vi "Setup file output channels.vi"(8 "error in":errorcluster, 9 "Sampling data":T1 {"Channels"."Hi cutoff" items=["500"=500.0, "1k"=1000.0, "5k"=5000.0, "10k"=10000.0, "20k"=20000.0]; "Channels"."Lo cutoff" items=["0.1"=0.1, "1"=1.0, "10"=10.0, "100"=100.0, "300"=300.0]; "Channels"."Gain" items=["x100"=100, "x1000"=1000, "x10000"=10000]}, 11 "file ref in":T3 format="%.0x") -> (0 "error out":errorcluster, 1 "Sampling data out":T1 {"Channels"."Hi cutoff" items=["500"=500.0, "1k"=1000.0, "5k"=5000.0, "10k"=10000.0, "20k"=20000.0]; "Channels"."Lo cutoff" items=["0.1"=0.1, "1"=1.0, "10"=10.0, "100"=100.0, "300"=300.0]; "Channels"."Gain" items=["x100"=100, "x1000"=1000, "x10000"=10000]}, 2 "dset ref":i32, 3 "file ref out":T3 format="%.0x", 4 "cmd dset out":i32)   [LabVIEW 2012]
uses:
  <vilib>/addons/h5labview2/base/hid_t.ctl
  Sampling info.ctl
  Channel.ctl
  Create HDF5 chunked dataset (2D).vi
  <vilib>/addons/h5labview2/base/H5Equery.vi
  <vilib>/addons/h5labview2/attrib/H5Awrite.llb/H5Awrite.xnode
  <vilib>/addons/h5labview2/group/H5G.lvlib
  <vilib>/addons/h5labview2/h5labview32.dll
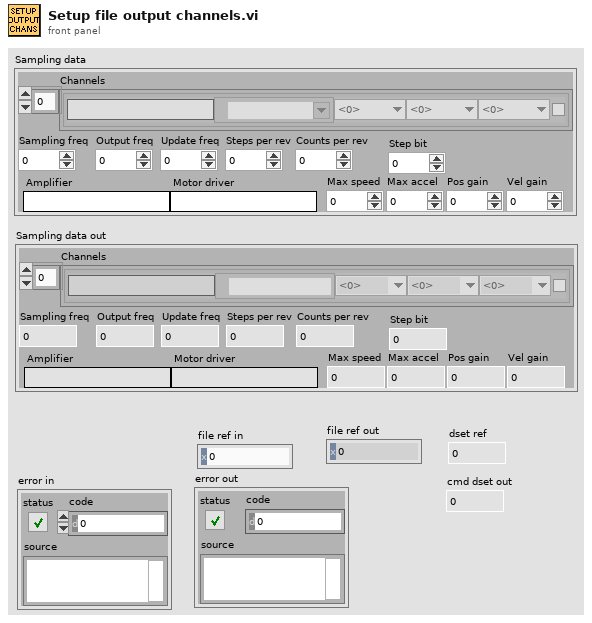
[diagram p1: front panel]
types:
  T1 = typedef "Sampling info.ctl" = cluster{"Channels":T2[], "Sampling freq":i32, "Output freq":i32, "Update freq":i32, "Steps per rev":i32, "Counts per rev":i32, "Amplifier":string, "Motor driver":string, "Step bit":u8, "Max speed":dbl, "Max accel":dbl, "Pos gain":dbl, "Vel gain":dbl}
  T2 = typedef "Channel.ctl" = cluster{"Name":string, "Chan":tag, "Gain":u16, "Lo cutoff":dbl, "Hi cutoff":dbl, "Notch":bool}
  T3 = typedef "hid_t.ctl" = i32
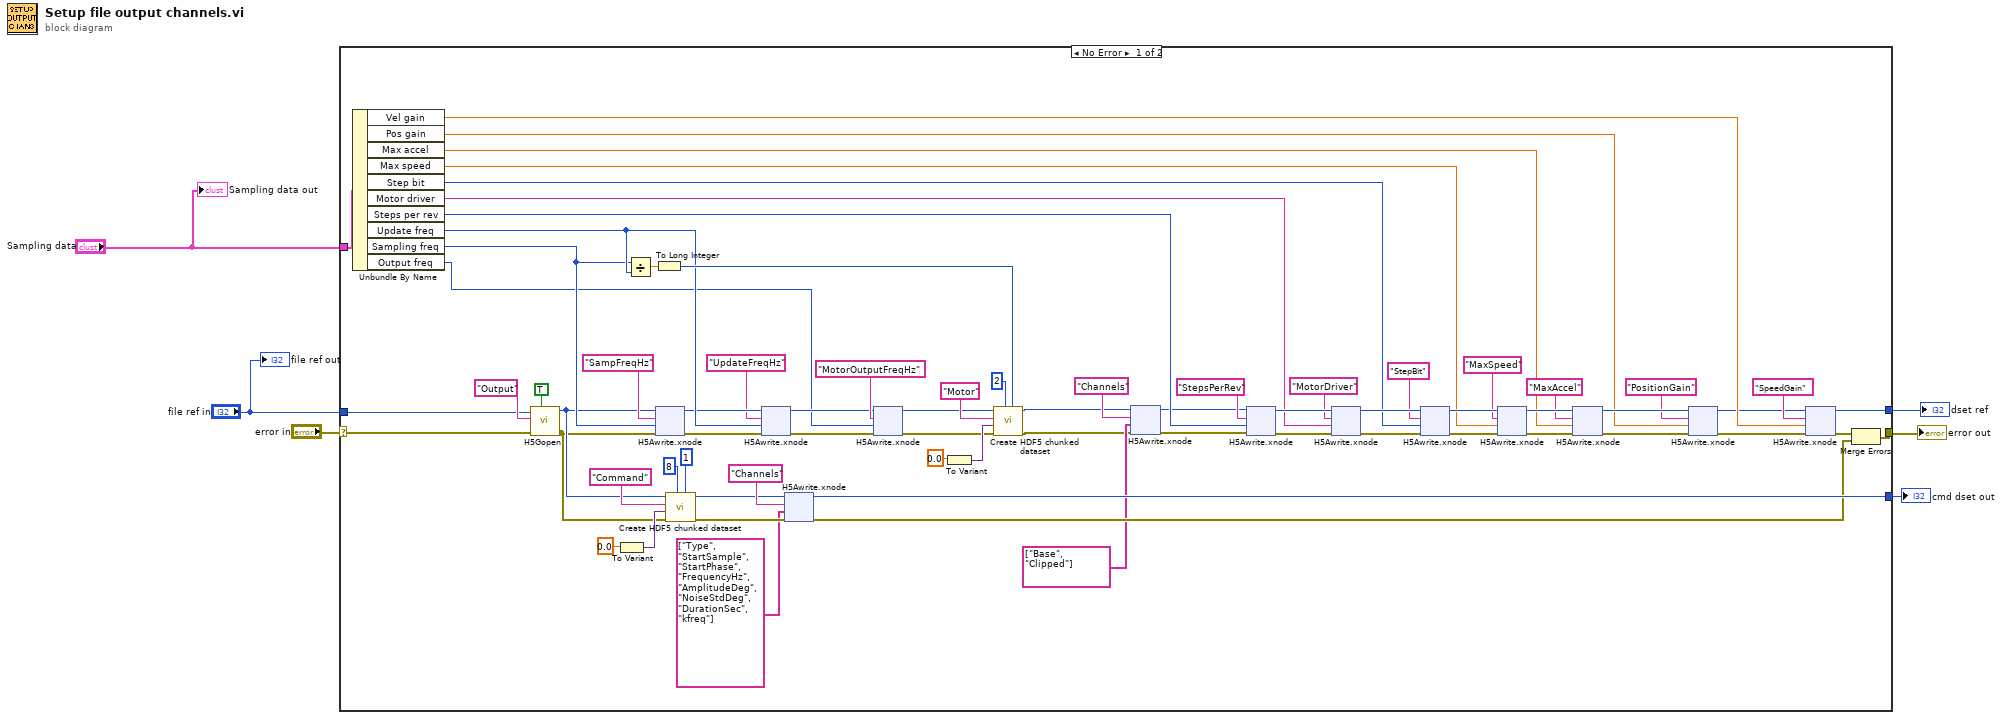
[diagram p0: block diagram]
diagram:
  n1 = case shown="No Error" "error in" {
    selector: "error in" -> [w47 w282]
    tunnel: [w29 _] -> w6
    tunnel: [w14 w282] -> w5
    tunnel: "file ref in" -> [w46 _]
    tunnel: "Sampling data" -> [w65 _]
    tunnel: [w16 _] -> w1
    frame No Error {
      n2 = Unbundle By Name(w65) -> ("Vel gain"=w32:dbl, "Pos gain"=w34:dbl, "Max accel"=w35:dbl, "Max speed"=w36:dbl, "Step bit"=w37:u8, "Motor driver"=w38:string, "Steps per rev"=w39:i32, "Update freq"=w62:i32, "Sampling freq"=w61:i32, "Output freq"=w42:i32)
      n3 = call <vilib>:"H5Gopen.vi"("create? (F)"=TRUE, "error in (no error)"=w47, "name"="Output", "ref in"=w46) -> ("error out"=w23:errorcluster, "group out"=w24:T3)  [unwired: 3 in]
      n4 = To Variant(anything=0.0) -> (Variant=w26:variant)
      n5 = Divide(x=w61, y=w62) -> (x/y=w63:dbl)
      n6 = To Long Integer(number=w63) -> (32bit integer=w64:i32)
      n7 = xnode "H5Awrite.xnode"("error in (no error)"=w23, "data"=w61, "attrib name"="SampFreqHz", "ref in"=w24) -> ("error out"=w55:errorcluster, "ref out"=w54:i32)  [unwired: 3 in, 1 out]
      n8 = call-poly "Create HDF5 chunked dataset.vi"("block size"=1, "number of channels"=8, "error in (no error)"=w23, "data type"=w26, "name"="Command", "ref in"=w24) -> ("error out"=w19:errorcluster, "dset out"=w20:i32)  [unwired: 4 in]
      n9 = xnode "H5Awrite.xnode"("error in (no error)"=w55, "data"=w62, "attrib name"="UpdateFreqHz", "ref in"=w54) -> ("error out"=w43:errorcluster, "ref out"=w44:i32)  [unwired: 3 in, 1 out]
      n10 = xnode "H5Awrite.xnode"("error in (no error)"=w19, "data"=string[] ["Type", "StartSample", "StartPhase", "FrequencyHz", "AmplitudeDeg", "NoiseStdDeg", "DurationSec", "kfreq"], "attrib name"="Channels", "ref in"=w20) -> ("error out"=w13:errorcluster, "ref out"=w16:i32)  [unwired: 3 in, 1 out]
      n11 = xnode "H5Awrite.xnode"("error in (no error)"=w43, "data"=w42, "attrib name"="MotorOutputFreqHz", "ref in"=w44) -> ("error out"=w40:errorcluster, "ref out"=w41:i32)  [unwired: 3 in, 1 out]
      n12 = To Variant(anything=0.0) -> (Variant=w48:variant)
      n13 = call-poly "Create HDF5 chunked dataset.vi"("block size"=w64, "number of channels"=2, "error in (no error)"=w40, "data type"=w48, "name"="Motor", "ref in"=w41) -> ("error out"=w9:errorcluster, "dset out"=w10:i32)  [unwired: 4 in]
      n14 = xnode "H5Awrite.xnode"("error in (no error)"=w9, "data"=string[] ["Base", "Clipped"], "attrib name"="Channels", "ref in"=w10) -> ("error out"=w7:errorcluster, "ref out"=w8:i32)  [unwired: 3 in, 1 out]
      n15 = xnode "H5Awrite.xnode"("error in (no error)"=w7, "data"=w39, "attrib name"="StepsPerRev", "ref in"=w8) -> ("error out"=w60:errorcluster, "ref out"=w59:i32)  [unwired: 3 in, 1 out]
      n16 = xnode "H5Awrite.xnode"("error in (no error)"=w60, "data"=w38, "attrib name"="MotorDriver", "ref in"=w59) -> ("error out"=w71:errorcluster, "ref out"=w70:T3)  [unwired: 3 in, 1 out]
      n17 = xnode "H5Awrite.xnode"("error in (no error)"=w71, "data"=w37, "attrib name"="StepBit", "ref in"=w70) -> ("error out"=w73:errorcluster, "ref out"=w72:T3)  [unwired: 3 in, 1 out]
      n18 = xnode "H5Awrite.xnode"("error in (no error)"=w73, "data"=w36, "attrib name"="MaxSpeed", "ref in"=w72) -> ("error out"=w75:errorcluster, "ref out"=w74:T3)  [unwired: 3 in, 1 out]
      n19 = xnode "H5Awrite.xnode"("error in (no error)"=w75, "data"=w35, "attrib name"="MaxAccel", "ref in"=w74) -> ("error out"=w76:errorcluster, "ref out"=w77:T3)  [unwired: 3 in, 1 out]
      n20 = xnode "H5Awrite.xnode"("error in (no error)"=w76, "data"=w34, "attrib name"="PositionGain", "ref in"=w77) -> ("error out"=w31:errorcluster, "ref out"=w30:T3)  [unwired: 3 in, 1 out]
      n21 = xnode "H5Awrite.xnode"("error in (no error)"=w31, "data"=w32, "attrib name"="SpeedGain", "ref in"=w30) -> ("error out"=w15:errorcluster, "ref out"=w29:T3)  [unwired: 3 in, 1 out]
      n22 = Merge Errors(w15, w13) -> (w14:errorcluster)
    }
    frame Error {
    }
  }
  "dset ref" <- w6
  "error out" <- w5
  "cmd dset out" <- w1
  "file ref out" <- "file ref in"
  "Sampling data out" <- "Sampling data"
